vi "Close.vi"(8 "error in (no error)":errorcluster, 11 "IV_meas in":refnum<class "IV_meas.lvclass">) -> (0 "error out":errorcluster, 3 "IV_meas out":refnum<class "IV_meas.lvclass">)   [LabVIEW 2014, in "IV_meas.lvclass"]
uses:
  IV_meas.lvclass
  Abstract/Instrument/Instrument/Instrument.lvclass
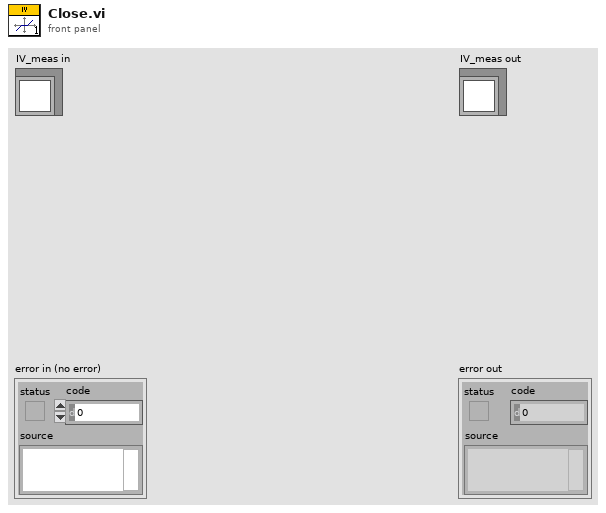
[diagram p1: front panel]
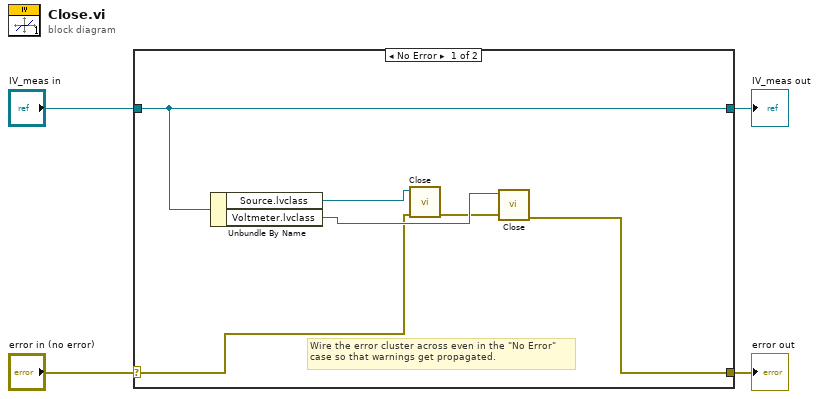
[diagram p0: block diagram]
diagram:
  n1 = case shown="No Error" "error in (no error)" {
    selector: "error in (no error)" -> [w6 w12]
    tunnel: [w5 w12] -> w3
    tunnel: [w7 w11] -> w1
    tunnel: "IV_meas in" -> [w7 w11]
    frame No Error {
      # "Wire the error cluster across even in the \"No Error\"\ncase so that warnings get propagated."
      n2 = Unbundle By Name(w7) -> ("Source.lvclass"=w10:refnum<class "Instrument.lvclass">, "Voltmeter.lvclass"=w9:refnum<class "Instrument.lvclass">)
      n3 = call-dynamic "Close.vi"("error in (no error)"=w6, "Instrument in"=w10) -> ("error out"=w8:errorcluster)  [unwired: 8 in, 1 out]
      n4 = call-dynamic "Close.vi"("error in (no error)"=w8, "Instrument in"=w9) -> ("error out"=w5:errorcluster)  [unwired: 8 in, 1 out]
    }
    frame Error {
    }
  }
  "error out" <- w3
  "IV_meas out" <- w1
